vi "Image procession FPGA-peek.vi"() -> ()   [LabVIEW 2016]
uses:
  <vilib>/visionFPGA/Controls/IMAQ FPGA Image Size.ctl
  <vilib>/rvi/Emulation/niFpgaSctlEmulationGetInTimedLoop.vi
  <vilib>/rvi/Emulation/niFpgaProcessEmulError.vi
  <vilib>/rvi/Emulation/niFpgaGetClockAttributes.vi
  <vilib>/rvi/Emulation/niFpgaEmulationReportErrorSimple.vi
  <vilib>/visionFPGA/Basics/FIFO to Pixel Bus/IMAQ FPGA FIFO to Pixel Bus RGB32x1.vi
  <vilib>/rvi/Emulation/niFpgaCriticalErrorInLSC.vi
  <vilib>/visionFPGA/NI_VDM_FPGA_Basics.lvlib
panel:
  in  "Image Size 3":T1={"Width"=640, "Height"=480}
  out "Output Valid 3":bool
  out "Output Valid 2":bool
  in  "Image Size 2":T1={"Width"=640, "Height"=480}
  out "Ready For Output3":bool=TRUE
  out "StartOfImage3":bool=TRUE
  out "Ready For Output2":bool=TRUE
  out "StartOfImage2":bool=TRUE
  out "Output Valid":bool
  out "Ready For Output1":bool=TRUE
  out "StartOfImage1":bool=TRUE
  in  "Image Size":T1={"Width"=640, "Height"=480}
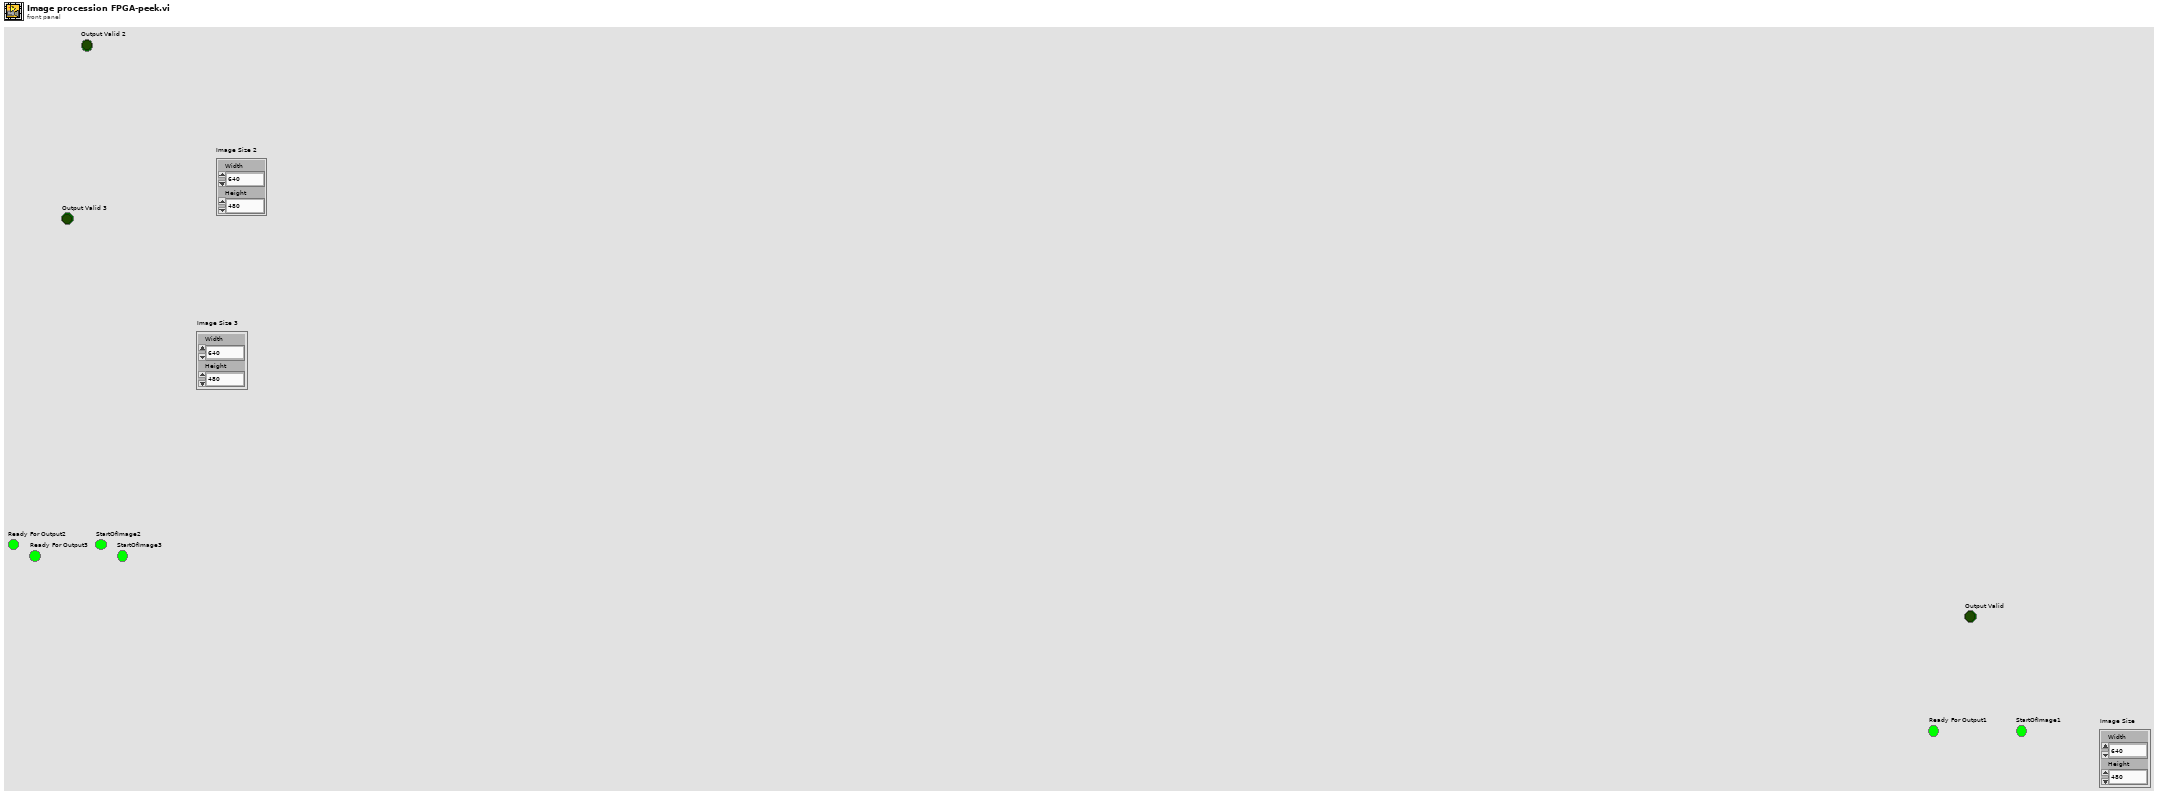
[diagram p1: front panel]
types:
  T1 = typedef "IMAQ FPGA Image Size.ctl" = cluster{"Width":u32, "Height":u32}
  T2 = typedef "IMAQ FPGA Pixel Bus RGB32x1.ctl" = cluster{"Pixel Data":cluster{"A":u8, "R/H":u8, "G/S":u8, "B/L":u8}, "DV":bool, "EOL":bool, "EOI":bool, "Data Type":enum16{"RGB32 x 1"}}
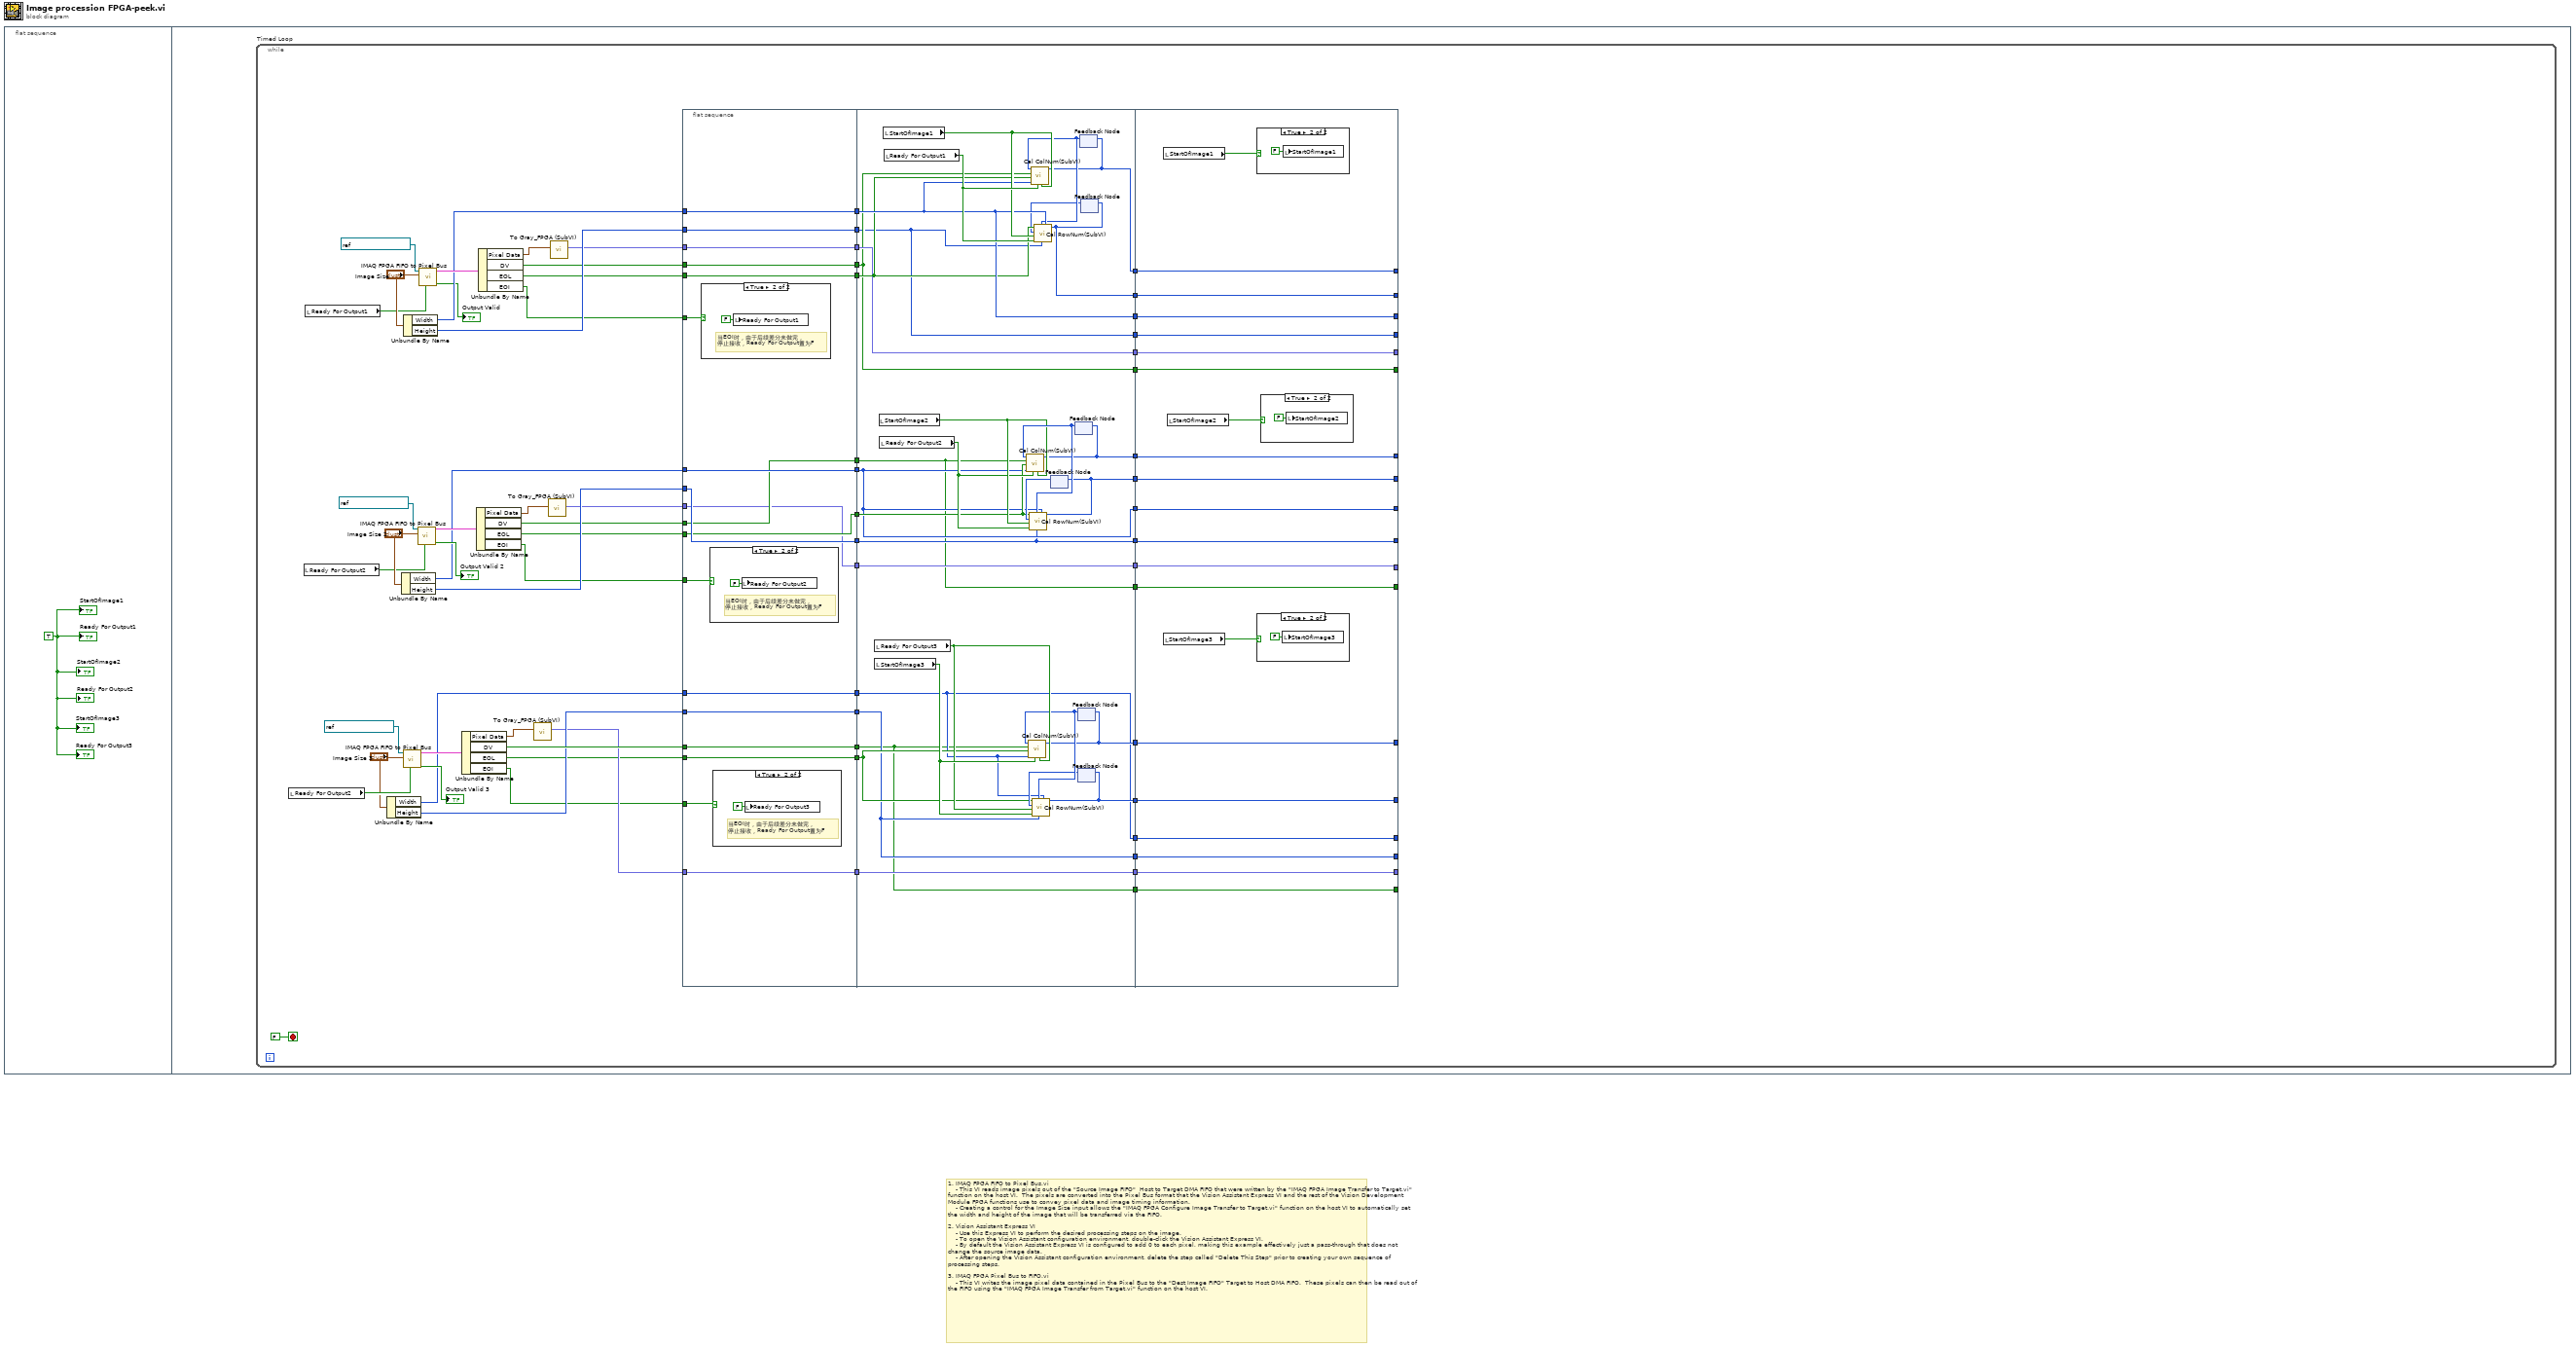
[diagram p0: block diagram]
diagram:
  # "1. IMAQ FPGA FIFO to Pixel Bus.vi\n    - This VI reads image pixels out of the \"Source Image FIFO\"  Host to Target DMA FIFO that were written by the \"IMAQ FPGA Image Transfer to Target.vi\" function on the host VI.  The pixels are converted into the Pixel Bus format that the Vision Assistant Express VI and the rest of the Vision Development Module FPGA functions use to convey pixel data and image timing information.\n    - Creating a control for the Image Size input allows the \"IMAQ FPGA Configure Image Transfer to Target.vi\" function on the host VI to automatically set the width and height of the image that will be transferred via the FIFO.\n\n2. Vision Assistant Express VI\n    - Use this Express VI to perform the desired processing steps on the image.\n    - To open the Vision Assistant configuration environment, double-click the Vision Assistant Express VI.\n    - By default the Vision Assistant Express VI is configured to add 0 to each pixel, making this example effectively just a pass-through that does not change the source image data.\n    - After opening the Vision Assistant configuration environment, delete the step called \"Delete This Step\" prior to creating your own sequence of processing steps.\n\n3. IMAQ FPGA Pixel Bus to FIFO.vi\n    - This VI writes the image pixel data contained in the Pixel Bus to the \"Dest Image FIFO\" Target to Host DMA FIFO.  These pixels can then be read out of the FIFO using the \"IMAQ FPGA Image Transfer from Target.vi\" function on the host VI."
  n1 = flat-sequence {
    frame #0 {
      w1 = TRUE ("Ready For Output")
      "StartOfImage1" <- w1
      "Ready For Output1" <- w1
      "StartOfImage2" <- w1
      "Ready For Output2" <- w1
      "StartOfImage3" <- w1
      "Ready For Output3" <- w1
    }
    frame #1 {
      n2 = while "Timed Loop" {
        stop <- FALSE stop-if-true
        n3 = local read "Ready For Output2"() -> (w22:bool)
        n4 = local read "Ready For Output2"() -> (w44:bool)
        n5 = local read "Ready For Output1"() -> (w58:bool)
        n6 = Unbundle By Name("Image Size 3") -> ("Width"=w16:u32, "Height"=w15:u32)
        n7 = Unbundle By Name("Image Size 2") -> ("Width"=w41:u32, "Height"=w40:u32)
        n8 = Unbundle By Name("Image Size") -> ("Width"=w66:u32, "Height"=w68:u32)
        n9 = call-poly <vilib>:"IMAQ FPGA FIFO to Pixel Bus.vi"("Ready For Output"=w22, "Image Size"="Image Size 3", "Source Image FIFO"=refnum<k21> "32it Source FIFO") -> ("Output Valid"=→"Output Valid 3":bool, "Pixel Bus Out"=w20:T2)  [unwired: 6 in, 1 out]
        n10 = call-poly <vilib>:"IMAQ FPGA FIFO to Pixel Bus.vi"("Ready For Output"=w44, "Image Size"="Image Size 2", "Source Image FIFO"=refnum<k21> "32it Source FIFO") -> ("Output Valid"=→"Output Valid 2":bool, "Pixel Bus Out"=w46:T2)  [unwired: 6 in, 1 out]
        n11 = call-poly <vilib>:"IMAQ FPGA FIFO to Pixel Bus.vi"("Ready For Output"=w58, "Image Size"="Image Size", "Source Image FIFO"=refnum<k21> "32it Source FIFO") -> ("Output Valid"=→"Output Valid":bool, "Pixel Bus Out"=w70:T2)  [unwired: 6 in, 1 out]
        n12 = Unbundle By Name(w20) -> ("Pixel Data"=w24:cluster{"A":u8, "R/H":u8, "G/S":u8, "B/L":u8}, "DV"=w18:bool, "EOL"=w13:bool, "EOI"=w12:bool)
        n13 = Unbundle By Name(w46) -> ("Pixel Data"=w42:cluster{"A":u8, "R/H":u8, "G/S":u8, "B/L":u8}, "DV"=w38:bool, "EOL"=w37:bool, "EOI"=w36:bool)
        n14 = Unbundle By Name(w70) -> ("Pixel Data"=w49:cluster{"A":u8, "R/H":u8, "G/S":u8, "B/L":u8}, "DV"=w48:bool, "EOL"=w59:bool, "EOI"=w67:bool)
        n15 = call "To Gray_FPGA (SubVI).vi"("Pixel Data"=w24) -> ("Data Out"=w14:fxp<+,8,8>)  [unwired: 10 in]
        n16 = call "To Gray_FPGA (SubVI).vi"("Pixel Data"=w42) -> ("Data Out"=w39:fxp<+,8,8>)  [unwired: 10 in]
        n17 = call "To Gray_FPGA (SubVI).vi"("Pixel Data"=w49) -> ("Data Out"=w50:fxp<+,8,8>)  [unwired: 10 in]
        n18 = flat-sequence {
          tunnel: w59 -> [w85]
          tunnel: w67 -> [w84]
          tunnel: w48 -> [w86]
          tunnel: w68 -> [w87]
          tunnel: w66 -> [w88]
          tunnel: w50 -> [w89]
          tunnel: [w89] -> w57
          tunnel: [w88] -> w56
          tunnel: [w87] -> w55
          tunnel: [w86] -> w54
          tunnel: [w85] -> w53
          tunnel: w41 -> [w82]
          tunnel: w40 -> [w81]
          tunnel: w39 -> [w78]
          tunnel: w38 -> [w80]
          tunnel: w37 -> [w79]
          tunnel: w36 -> [w83]
          tunnel: [w82] -> w35
          tunnel: [w81] -> w34
          tunnel: [w80] -> w33
          tunnel: [w79] -> w32
          tunnel: [w78] -> w26
          tunnel: w18 -> [w77]
          tunnel: [w77] -> w17
          tunnel: w16 -> [w76]
          tunnel: w15 -> [w75]
          tunnel: w14 -> [w72]
          tunnel: w13 -> [w74]
          tunnel: w12 -> [w73]
          tunnel: [w76] -> w11
          tunnel: [w75] -> w10
          tunnel: [w74] -> w9
          tunnel: [w72] -> w3
          tunnel: [w117] -> w65
          tunnel: [w115] -> w64
          tunnel: [w125] -> w63
          tunnel: [w122] -> w62
          tunnel: [w119] -> w61
          tunnel: [w120] -> w60
          tunnel: w57 -> [w125]
          tunnel: w56 -> [w122]
          tunnel: w55 -> [w119]
          tunnel: w54 -> [w120]
          tunnel: w53 -> [w121]
          tunnel: w35 -> [w103]
          tunnel: w34 -> [w102]
          tunnel: w33 -> [w100]
          tunnel: w32 -> [w106]
          tunnel: [w105] -> w31
          tunnel: [w104] -> w30
          tunnel: [w103] -> w29
          tunnel: [w102] -> w28
          tunnel: [w101] -> w27
          tunnel: w26 -> [w101]
          tunnel: [w100] -> w25
          tunnel: w17 -> [w93]
          tunnel: w11 -> [w96]
          tunnel: w10 -> [w95]
          tunnel: w9 -> [w99]
          tunnel: [w98] -> w8
          tunnel: [w97] -> w7
          tunnel: [w96] -> w6
          tunnel: [w95] -> w5
          tunnel: [w94] -> w4
          tunnel: w3 -> [w94]
          tunnel: [w93] -> w2
          tunnel: w65 -> [w140]
          tunnel: w64 -> [w141]
          tunnel: w63 -> [w137]
          tunnel: w62 -> [w139]
          tunnel: w61 -> [w138]
          tunnel: w60 -> [w144]
          tunnel: w31 -> [w143]
          tunnel: w30 -> [w136]
          tunnel: w29 -> [w135]
          tunnel: w28 -> [w134]
          tunnel: w27 -> [w133]
          tunnel: w25 -> [w132]
          tunnel: [w144] -> _
          tunnel: [w143] -> _
          tunnel: [w141] -> _
          tunnel: [w140] -> _
          tunnel: [w139] -> _
          tunnel: [w138] -> _
          tunnel: [w137] -> _
          tunnel: [w136] -> _
          tunnel: [w135] -> _
          tunnel: [w134] -> _
          tunnel: [w133] -> _
          tunnel: [w132] -> _
          tunnel: [w131] -> _
          tunnel: w8 -> [w131]
          tunnel: [w130] -> _
          tunnel: w7 -> [w130]
          tunnel: w6 -> [w129]
          tunnel: w5 -> [w128]
          tunnel: w4 -> [w127]
          tunnel: w2 -> [w126]
          tunnel: [w129] -> _
          tunnel: [w128] -> _
          tunnel: [w127] -> _
          tunnel: [w126] -> _
          frame #0 {
            n19 = case shown="True" w84 {
              frame False {
              }
              frame True {
                # "当EOI时，由于后续差分未做完，\n停止接收，Ready For Output置为F"
                n20 = local write "Ready For Output1"(FALSE ("Ready For Output")) -> ()
              }
            }
            n21 = case shown="True" w83 {
              frame False {
              }
              frame True {
                # "当EOI时，由于后续差分未做完，\n停止接收，Ready For Output置为F"
                n22 = local write "Ready For Output2"(FALSE ("Ready For Output")) -> ()
              }
            }
            n23 = case shown="True" w73 {
              frame False {
              }
              frame True {
                # "当EOI时，由于后续差分未做完，\n停止接收，Ready For Output置为F"
                n24 = local write "Ready For Output3"(FALSE ("Ready For Output")) -> ()
              }
            }
          }
          frame #1 {
            n25 = local read "Ready For Output3"() -> (w109:bool)
            n26 = local read "StartOfImage3"() -> (w110:bool)
            n27 = local read "StartOfImage2"() -> (w112:bool)
            n28 = local read "Ready For Output2"() -> (w111:bool)
            n29 = local read "StartOfImage1"() -> (w123:bool)
            n30 = local read "Ready For Output1"() -> (w124:bool)
            n31 = feedback #1() -> (w114:u16)  [unwired: 1 in]
            n32 = feedback #2() -> (w113:u16)  [unwired: 1 in]
            n33 = call "Cal ColNum(SubVI).vi"("StartOfImage"=w112, "Ready For Input"=w111, "Width"=w103, "EOL"=w106, "DV"=w100, "curColNum"=w113) -> ("nextColNum"=w105:u16)  [unwired: 5 in]
            n34 = call "Cal RowNum(SubVI).vi"("Width"=w103, "Height"=w102, "curCol"=w113, "Ready For Input"=w111, "startOfImage"=w112, "curRow"=w114, "EOL"=w106) -> ("nextRow"=w104:u16)  [unwired: 4 in]
            n35 = feedback-in #1(w104) -> ()
            n36 = feedback-in #2(w105) -> ()
            n37 = feedback #3() -> (w108:u16)  [unwired: 1 in]
            n38 = call "Cal ColNum(SubVI).vi"("StartOfImage"=w109, "Ready For Input"=w110, "Width"=w96, "EOL"=w99, "DV"=w93, "curColNum"=w108) -> ("nextColNum"=w98:u16)  [unwired: 5 in]
            n39 = feedback-in #3(w98) -> ()
            n40 = feedback #4() -> (w107:u16)  [unwired: 1 in]
            n41 = call "Cal RowNum(SubVI).vi"("Width"=w96, "Height"=w95, "curCol"=w108, "Ready For Input"=w110, "startOfImage"=w109, "curRow"=w107, "EOL"=w99) -> ("nextRow"=w97:u16)  [unwired: 4 in]
            n42 = feedback-in #4(w97) -> ()
            n43 = feedback #5() -> (w118:u16)  [unwired: 1 in]
            n44 = call "Cal ColNum(SubVI).vi"("StartOfImage"=w123, "Ready For Input"=w124, "Width"=w122, "EOL"=w121, "DV"=w120, "curColNum"=w118) -> ("nextColNum"=w115:u16)  [unwired: 5 in]
            n45 = feedback-in #5(w115) -> ()
            n46 = feedback #6() -> (w116:u16)  [unwired: 1 in]
            n47 = call "Cal RowNum(SubVI).vi"("Width"=w122, "Height"=w119, "curCol"=w118, "Ready For Input"=w124, "startOfImage"=w123, "curRow"=w116, "EOL"=w121) -> ("nextRow"=w117:u16)  [unwired: 4 in]
            n48 = feedback-in #6(w117) -> ()
          }
          frame #2 {
            n49 = local read "StartOfImage3"() -> (w142:bool)
            n50 = local read "StartOfImage1"() -> (w146:bool)
            n51 = local read "StartOfImage2"() -> (w145:bool)
            n52 = case shown="True" w142 {
              frame False {
              }
              frame True {
                n53 = local write "StartOfImage3"(FALSE ("StartOfImage")) -> ()
              }
            }
            n54 = case shown="True" w146 {
              frame False {
              }
              frame True {
                n55 = local write "StartOfImage1"(FALSE ("StartOfImage")) -> ()
              }
            }
            n56 = case shown="True" w145 {
              frame False {
              }
              frame True {
                n57 = local write "StartOfImage2"(FALSE ("StartOfImage")) -> ()
              }
            }
          }
        }
      }
    }
  }
